vi "Decimate plate middles.vi"(5 "Decimate Factor (5)":i32=5, 7 "Points in rim (10)":i32=10, 9 "Heights [array] (mm) in":dbl[](array[numeric]), 10 "dY[array] (mm) in":dbl[](array[numeric]), 11 "X[array] (mm) in":dbl[](array[numeric])) -> (1 "Heights [array] (mm) decimated out":dbl[](array[numeric]), 2 "dY[array] (mm) decimated out":dbl[](array[numeric]), 3 "X[array] (mm) decimated out":dbl[](array[numeric]))   [LabVIEW 2009]
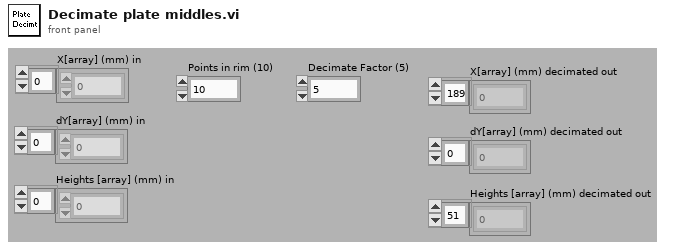
[diagram p1: front panel]
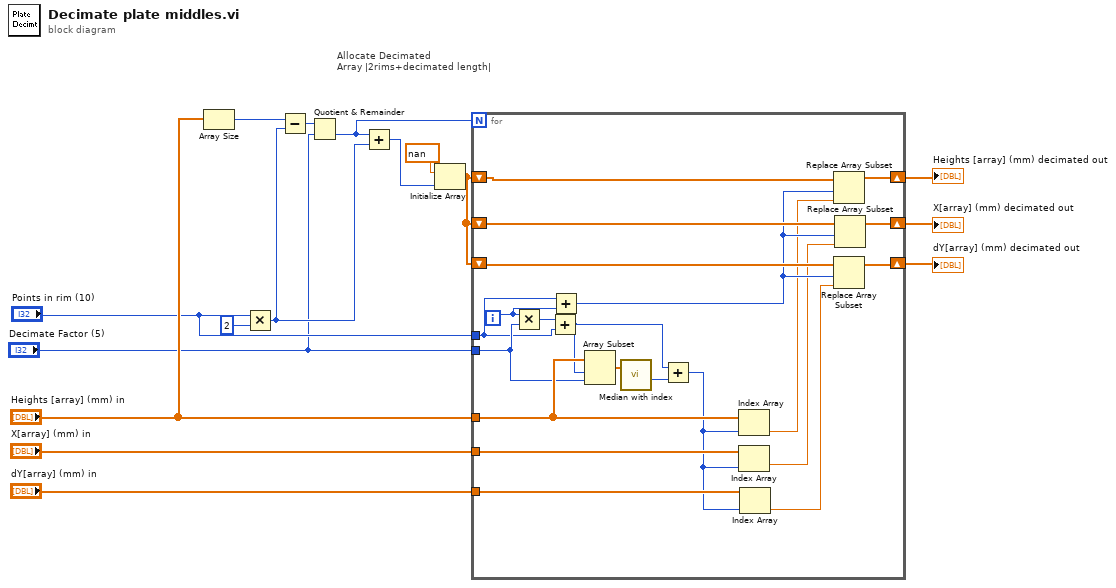
[diagram p0: block diagram]
diagram:
  # "Allocate Decimated\nArray |2rims+decimated length|"
  n1 = Array Size(array="Heights [array] (mm) in") -> (size(s)=w14:i32)
  n2 = Multiply(x="Points in rim (10)", y=2) -> (x*y=w13:i32)
  n3 = Subtract(x=w14, y=w13) -> (x-y=w15:i32)
  n4 = Quotient & Remainder(x=w15, y="Decimate Factor (5)") -> (floor(x/y)=w10:i32)  [unwired: 1 out]
  n5 = Add(x=w10, y=w13) -> (x+y=w8:i32)
  n6 = Initialize Array(nan ("element"), w8) -> (w4:dbl[])
  n7 = for {
    N: w10 -> [_]
    tunnel: "Heights [array] (mm) in" -> [w37]
    tunnel: "Points in rim (10)" -> [w29]
    tunnel: "Decimate Factor (5)" -> [w31]
    tunnel: "X[array] (mm) in" -> [w35]
    tunnel: "dY[array] (mm) in" -> [w34]
    shift-right: [w32] -> w3
    shift-left: w4 -> [w33]
    shift-right: [w23] -> w2
    shift-left: w4 -> [w27]
    shift-right: [w26] -> w1
    shift-left: w4 -> [w25]
    i -> [w30]
    n8 = Multiply(x=w30, y=w31) -> (x*y=w28:i32)
    n9 = Add(x=w28, y=w29) -> (x+y=w18:i32)
    n10 = Add(x=w29, y=w30) -> (x+y=w24:i32)
    n11 = Array Subset(array=w37, index=w18, length=w31) -> (w36:dbl[])
    n12 = call "Median with index.vi"("Data in"=w36) -> ("Median Index"=w19:i32)  [unwired: 9 in, 1 out]
    n13 = Add(x=w18, y=w19) -> (x+y=w17:i32)
    n14 = Index Array(array=w37, index=w17) -> (element=w22:dbl)
    n15 = Index Array(array=w35, index=w17) -> (element=w21:dbl)
    n16 = Index Array(array=w34, index=w17) -> (element=w20:dbl)
    n17 = Replace Array Subset(array=w33, new element=w22, index=w24) -> (w32:dbl[])
    n18 = Replace Array Subset(array=w25, new element=w20, index=w24) -> (w26:dbl[])
    n19 = Replace Array Subset(array=w27, new element=w21, index=w24) -> (w23:dbl[])
  }
  "Heights [array] (mm) decimated out" <- w3
  "X[array] (mm) decimated out" <- w2
  "dY[array] (mm) decimated out" <- w1
